vi "hamamatsu_test_global.vi"() -> ()   [LabVIEW 2023]
panel:
  in  "Value in":dbl=5.0
  in  "Type":cluster{"Mode":u32, "Polarity":u32}={"Mode"=1, "Polarity"=1} {"Polarity" items=["Negative"=1, "Positive"=2]; "Mode" items=["Low"=1, "Global Exposure"=2, "Programmable"=3, "Trigger Ready"=4, "High"=5]}
  in  "Programmable Options":cluster{"Width":dbl, "Delay":dbl, "Source":u32}={"Width"=0.003, "Delay"=0.0, "Source"=2} {"Source" items=["Exposure"=1, "Readout End"=2, "V Sync"=3, "H Sync"=4, "Trigger"=6]}
  in  "Port":i32=1
  out "Current Frame Timestamp":dbl
  out "Image":u16[][](graph)
  in  "Play":bool
  in  "Acquire":bool
  out "Current Frame Index":i32=-1
  in  "Frames to Capture":i32=100
  out "Camera Serial":string
  out "Camera Model":string
  out "Camera Version":string
  out "Total Frames":i32
  out "error out":errorcluster {"code" format="%.0x"}
  in  "quit":bool
  # "This is an example of how to capture\ndata at full speed to RAM, then read \nthe data from the buffer later."
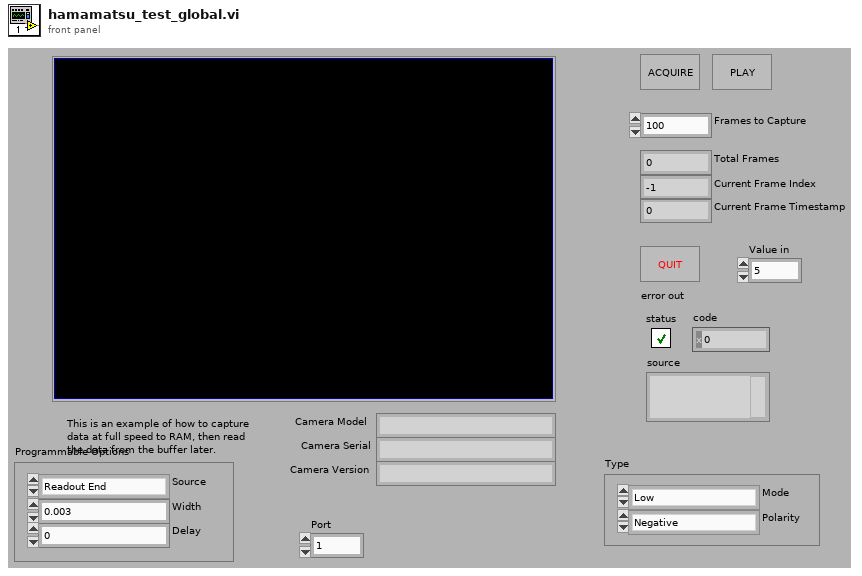
[diagram p1: front panel]
types:
  T1 = cluster{"Model":string, "Camera ID":string, "Firmware":string}
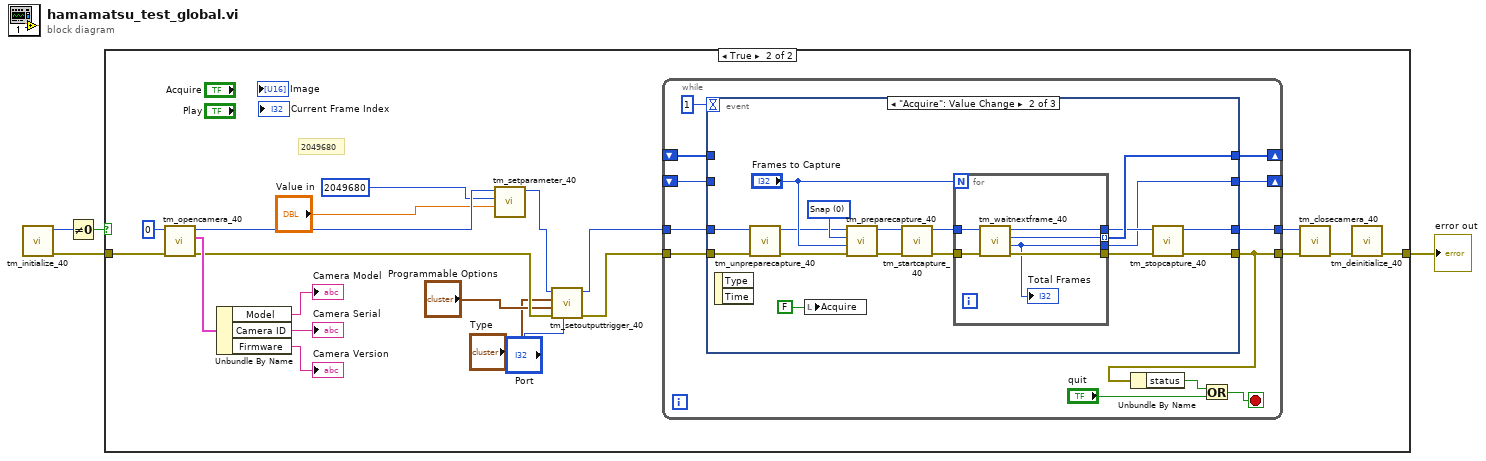
[diagram p0: block diagram]
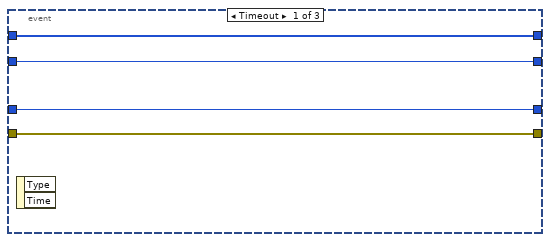
[diagram p3: hidden frame]
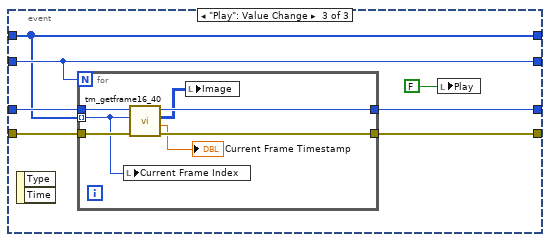
[diagram p4: hidden frame]
diagram:
  n1 = call <userlib>:"tm_initialize_40.vi"() -> ("error out"=w1:errorcluster, "Number Of Cameras"=w2:u32)  [unwired: 8 in, 2 out]
  n2 = Not Equal To 0?(x=w2) -> (x != 0?=w4:bool)
  n3 = case shown="True" w4 {
    tunnel: [w5 w22] -> w3
    tunnel: w1 -> [w5 w25]
    frame False {
    }
    frame True {
      # "2049680"
      n4 = call <userlib>:"tm_opencamera_40.vi"("error in (no error)"=w25, "Camera Index"=u32 0) -> ("error out"=w11:errorcluster, "Camera Details"=w19:T1, "Handle out"=w15:u32)  [unwired: 7 in]
      n5 = Unbundle By Name(w19) -> ("Model"=→"Camera Model":string, "Camera ID"=→"Camera Serial":string, "Firmware"=→"Camera Version":string)
      n6 = call <userlib>:"tm_setparameter_40.vi"("Value in"="Value in", "Parameter"=2049680 ("Frames to Capture 2"), "Handle in"=w15) -> ("Handle out"=w13:u32)  [unwired: 7 in, 1 out]
      n7 = call <userlib>:"tm_setoutputtrigger_40.vi"("Port"="Port", "error in (no error)"=w11, "Programmable Options"="Programmable Options", "Type"="Type", "Handle in"=w13) -> ("error out"=w10:errorcluster, "Handle out"=w12:u32)  [unwired: 5 in]
      n8 = while {
        tunnel: [w30] -> w21
        tunnel: [w37] -> w20
        tunnel: w12 -> [w35]
        tunnel: w10 -> [w34]
        shift-right: [w26] -> _
        shift-left: _ -> [w33]
        shift-right: [w32] -> _
        shift-left: _ -> [w31]
        stop <- w27 stop-if-true
        n9 = event shown="[1] \"Acquire\": Value Change" {
          selector: _ -> [_ _ _]
          dyn-events: _ -> [_ _ _]
          timeout: 1 -> [_ _ _]
          tunnel: [w40 w49 w71] -> w37
          tunnel: [w41 w50 w70] -> w30
          tunnel: w34 -> [w41 w45 w68]
          tunnel: w35 -> [w40 w42 w69]
          tunnel: [w38 w46 w67] -> w26
          tunnel: w33 -> [w38 _ w67]
          tunnel: [w39 w53 w65] -> w32
          tunnel: w31 -> [w39 _ w65]
          event Timeout {
            n10 = event-data() -> ()  [unwired: 1 in, 2 out]
          }
          event "Acquire": Value Change {
            w54 = 0 items=["Snap", "Sequence"] ("Capture mode")
            n11 = event-data() -> ()  [unwired: 1 in, 2 out]
            n12 = call <userlib>:"tm_unpreparecapture_40.vi"("error in (no error)"=w45, "Handle in"=w42) -> ("error out"=w44:errorcluster, "Handle out"=w43:u32)  [unwired: 8 in]
            n13 = local write "Acquire"(FALSE) -> ()
            n14 = call <userlib>:"tm_preparecapture_40.vi"("error in (no error)"=w44, "Frames"="Frames to Capture", "Capture mode"=w54, "Handle in"=w43) -> ("error out"=w55:errorcluster, "Handle out"=w56:u32)  [unwired: 4 in, 2 out]
            n15 = call <userlib>:"tm_startcapture_40.vi"("error in (no error)"=w55, "Handle in"=w56) -> ("error out"=w57:errorcluster, "Handle out"=w58:u32)  [unwired: 8 in]
            n16 = for {
              N: "Frames to Capture" -> [_]
              tunnel: w57 -> [w63]
              tunnel: w58 -> [w64]
              tunnel: [w61] -> w53 mode=indexing
              tunnel: [w62] -> w48
              tunnel: [w59] -> w46
              tunnel: [w60] -> w47
              n17 = call <userlib>:"tm_waitnextframe_40.vi"("error in (no error)"=w63, "Handle in"=w64) -> ("error out"=w60:errorcluster, "Frame Count"=w59:i32, "Frame Index"=w61:i32, "Handle out"=w62:u32)  [unwired: 6 in]
              "Total Frames" <- w59
            }
            n18 = call <userlib>:"tm_stopcapture_40.vi"("error in (no error)"=w47, "Handle in"=w48) -> ("error out"=w50:errorcluster, "Handle out"=w49:u32)  [unwired: 8 in]
          }
          event "Play": Value Change {
            n19 = event-data() -> ()  [unwired: 1 in, 2 out]
            n20 = for {
              N: w67 -> [_]
              tunnel: w65 -> [w73] mode=indexing
              tunnel: w68 -> [w78]
              tunnel: w69 -> [w77]
              tunnel: [w76] -> w70
              tunnel: [w75] -> w71
              n21 = local write "Current Frame Index"(w73) -> ()
              n22 = call <userlib>:"tm_getframe16_40.vi"("error in (no error)"=w78, "Frame Index"=w73, "Handle in"=w77) -> ("error out"=w76:errorcluster, "Timestamp"=→"Current Frame Timestamp":dbl, "Data"=w74:u16[][], "Handle out"=w75:u32)  [unwired: 5 in]
              n23 = local write "Image"(w74) -> ()
            }
            n24 = local write "Play"(FALSE) -> ()
          }
        }
        n25 = Unbundle By Name(w30) -> ("status"=w29:bool)
        n26 = Or(x=w29, y="quit") -> (x .or. y?=w27:bool)
      }
      n27 = call <userlib>:"tm_closecamera_40.vi"("error in (no error)"=w21, "Handle in"=w20) -> ("error out"=w23:errorcluster)  [unwired: 9 in]
      n28 = call <userlib>:"tm_deinitialize_40.vi"("error in (no error)"=w23) -> ("error out"=w22:errorcluster)  [unwired: 10 in]
    }
  }
  "error out" <- w3
